vi "Open Help.vi"(7 "CHM or HLP File Name":string="Eulogy.chm", 8 "Error In":errorcluster, 11 "HTML File Name":string="/pages/Add-on/Bookmark_Manager.html") -> (0 "Error Out":errorcluster)   [LabVIEW 2017, in "Bookmark Manager.lvlib"]
uses:
  Bookmark Manager.lvlib
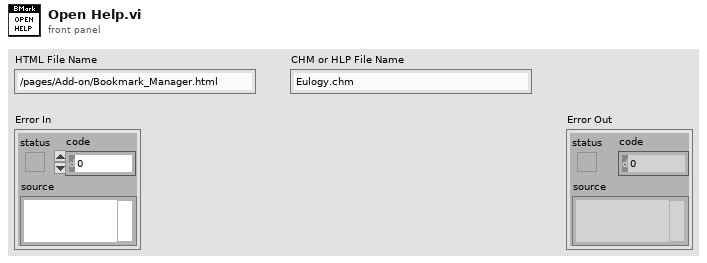
[diagram p1: front panel]
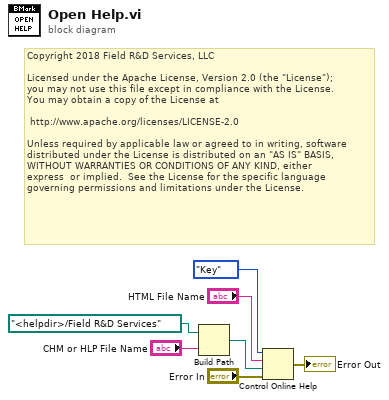
[diagram p0: block diagram]
diagram:
  # "Copyright 2018 Field R&D Services, LLC\n\nLicensed under the Apache License, Version 2.0 (the \"License\");\nyou may not use this file except in compliance with the License.\nYou may obtain a copy of the License at\n\n\thttp://www.apache.org/licenses/LICENSE-2.0\n\nUnless required by applicable law or agreed to in writing, software\ndistributed under the License is distributed on an \"AS IS\" BASIS,\nWITHOUT WARRANTIES OR CONDITIONS OF ANY KIND, either \nexpress  or implied.  See the License for the specific language \ngoverning permissions and limitations under the License."
  n1 = Build Path(base path=path "<helpdir>/Field R&D Services", name or relative path="CHM or HLP File Name") -> (appended path=w1:path)
  n2 = Control Online Help(1:"Error In", 2:w1, 3:"HTML File Name", 4:enum16{"Contents", "Key", "Close"}."Key" ("Operation")) -> (0:→"Error Out":errorcluster)
